vi "DiffDrivePoseEst_AddVisionMeasurement.vi"(9 "TImeStamp_Seconds":dbl=0.02, 10 "visionRobotPose":T10={"TRANSLATION"={"X"=0.0, "Y"=0.0}, "ROTATION"={"VALUE"=0.0, "COS"=1.0, "SIN"=0.0}} {"ROTATION"."SIN" format="%13.4f"; "ROTATION"."COS" format="%13.4f"; "ROTATION"."VALUE" format="%13.4f"; "TRANSLATION"."Y" format="%14.3f"; "TRANSLATION"."X" format="%14.3f"}, 11 "in DiffDrivePoseEstimate":T2={"M_VisionDiscR"=[], "m_nominal_dT"=0.0, "m_PrevTime_Sec"=0.0, "m_GyroOffset"={"VALUE"=0.0, "COS"=1.0, "SIN"=0.0}, "m_PrevAngle"={"VALUE"=0.0, "COS"=1.0, "SIN"=0.0}, "StartLeftEnc_M"=0.0, "StartRightEnc_M"=0.0, "m_Observer"={"m_P"=[], "m_xHat"=[], "States"=0, "Outputs"=0, "m_ContR"=[], "m_ContQ"=[], "m_SigmasF"=[], "m_dT_Sec"=0.0, "MERWE_SCALED_SIGMA_PTS"={"m_Wm"=[], "States"=0, "Alpha"=0.0, "m_Wc"=[], "Kappa"=0}, "meanFuncX"=refnum, "meanFuncY"=refnum, "residualFuncX"=refnum, "residualFuncY"=refnum, "addFuncX"=refnum, "addFuncXExtra"=variant, "residualFuncYExtra"=variant, "residualFuncXExtra"=variant, "MeanFuncYExtra"=variant, "MeanFuncXExtra"=variant, "Inputs"=0}, "m_latencyCompensator"={"m_pastObserverSnapshots "=[]}} {"m_PrevAngle"."SIN" format="%13.4f"; "m_PrevAngle"."COS" format="%13.4f"; "m_PrevAngle"."VALUE" format="%13.4f"; "m_GyroOffset"."SIN" format="%13.4f"; "m_GyroOffset"."COS" format="%13.4f"; "m_GyroOffset"."VALUE" format="%13.4f"}) -> (0 "Error":bool, 3 "Out DiffDrivePoseEstimate":T2={"M_VisionDiscR"=[], "m_nominal_dT"=0.0, "m_PrevTime_Sec"=0.0, "m_GyroOffset"={"VALUE"=0.0, "COS"=1.0, "SIN"=0.0}, "m_PrevAngle"={"VALUE"=0.0, "COS"=1.0, "SIN"=0.0}, "StartLeftEnc_M"=0.0, "StartRightEnc_M"=0.0, "m_Observer"={"m_P"=[], "m_xHat"=[], "States"=0, "Outputs"=0, "m_ContR"=[], "m_ContQ"=[], "m_SigmasF"=[], "m_dT_Sec"=0.0, "MERWE_SCALED_SIGMA_PTS"={"m_Wm"=[], "States"=0, "Alpha"=0.0, "m_Wc"=[], "Kappa"=0}, "meanFuncX"=refnum, "meanFuncY"=refnum, "residualFuncX"=refnum, "residualFuncY"=refnum, "addFuncX"=refnum, "addFuncXExtra"=variant, "residualFuncYExtra"=variant, "residualFuncXExtra"=variant, "MeanFuncYExtra"=variant, "MeanFuncXExtra"=variant, "Inputs"=0}, "m_latencyCompensator"={"m_pastObserverSnapshots "=[]}} {"m_PrevAngle"."SIN" format="%13.4f"; "m_PrevAngle"."COS" format="%13.4f"; "m_PrevAngle"."VALUE" format="%13.4f"; "m_GyroOffset"."SIN" format="%13.4f"; "m_GyroOffset"."COS" format="%13.4f"; "m_GyroOffset"."VALUE" format="%13.4f"})   [LabVIEW 2019, in "Trajectory_Library.lvlib"]
doc: "Add a vision measurement to the Unscented Kalman Filter. This will correct the odometry pose estimate while still accounting for measurement noise.\n \nThis method can be called as infrequently as you want, as long as you are calling DifferentialDrivePoseEstimator_update every loop.\n \nInputs:\n - InDIffDrivePoseEstimate -- Data cluster for this system\n - visionRobotPoseMeters -- The pose of the robot as measured by the vision camera.\n - timestampSeconds -- The timestamp of the vision measurement in seconds. Note that if you don't use your own time source by calling DifferentialDrivePoseEstimator_updateWithTime then you must use a timestamp with an epoch since FPGA startup (i.e. the epoch of this timestamp is the same epoch as Timer.getFPGATimestamp.) This means that you should use Timer.getFPGATimestamp as your time source in this case.\n\nOutputs:\n - OutDIffDrivePoseEstimate -- Data cluster for this system\n - Error -- Returns TRUE if an error occured."
uses:
  Trajectory_Library.lvlib
  DIFF_DRIVE_POSE_EST.ctl
  <vilib>/Analysis/Matrix/Datatypes/RealMatrix.ctl
  ROTATION2D.ctl
  UNSCENTED_KALMAN_FILTER.ctl
  MERWE_SCALED_SIGMA_PTS.ctl
  CALLBACK_FUNC_TYPE.ctl
  KALMAN_FILTER_LATENCY_COMP.ctl
  OBSERVER_SNAP_LIST_ITEM.ctl
  OBSERVER_SNAPSHOT.ctl
  POSE2D.ctl
  TRANSLATION2D.ctl
  VecBuilder_3x1Fill.vi
  Pose_getXYAngle.vi
  MatBuilder_Create.vi
  <vilib>/Analysis/Matrix/NI_Matrix.lvlib
panel:
  in  "Cluster":cluster{"VisionDiscreteR":T1}
  # "NOT A PARAMETER, JUST A DATA TYPE"
  # "<3, 3>"
  # "<Statess,1>"
  # "<States, States>"
  # "<Inputs, 1>"
  # "<Outputs,  1>"
  # "State Estimate <Statess,1>"
  # "<States, States>"
  # "<States, ?>"
  # "<Statess,  States>"
  # "<Outputs, Outputs>"
  # "<?, 1>"
  # "<?, 1>"
  # "<3, 3>"
  # "<Statess,1>"
  # "<States, States>"
  # "<Inputs, 1>"
  # "<Outputs,  1>"
  # "State Estimate <Statess,1>"
  # "<States, States>"
  # "<States, ?>"
  # "<Statess,  States>"
  # "<Outputs, Outputs>"
  # "<?, 1>"
  # "<?, 1>"
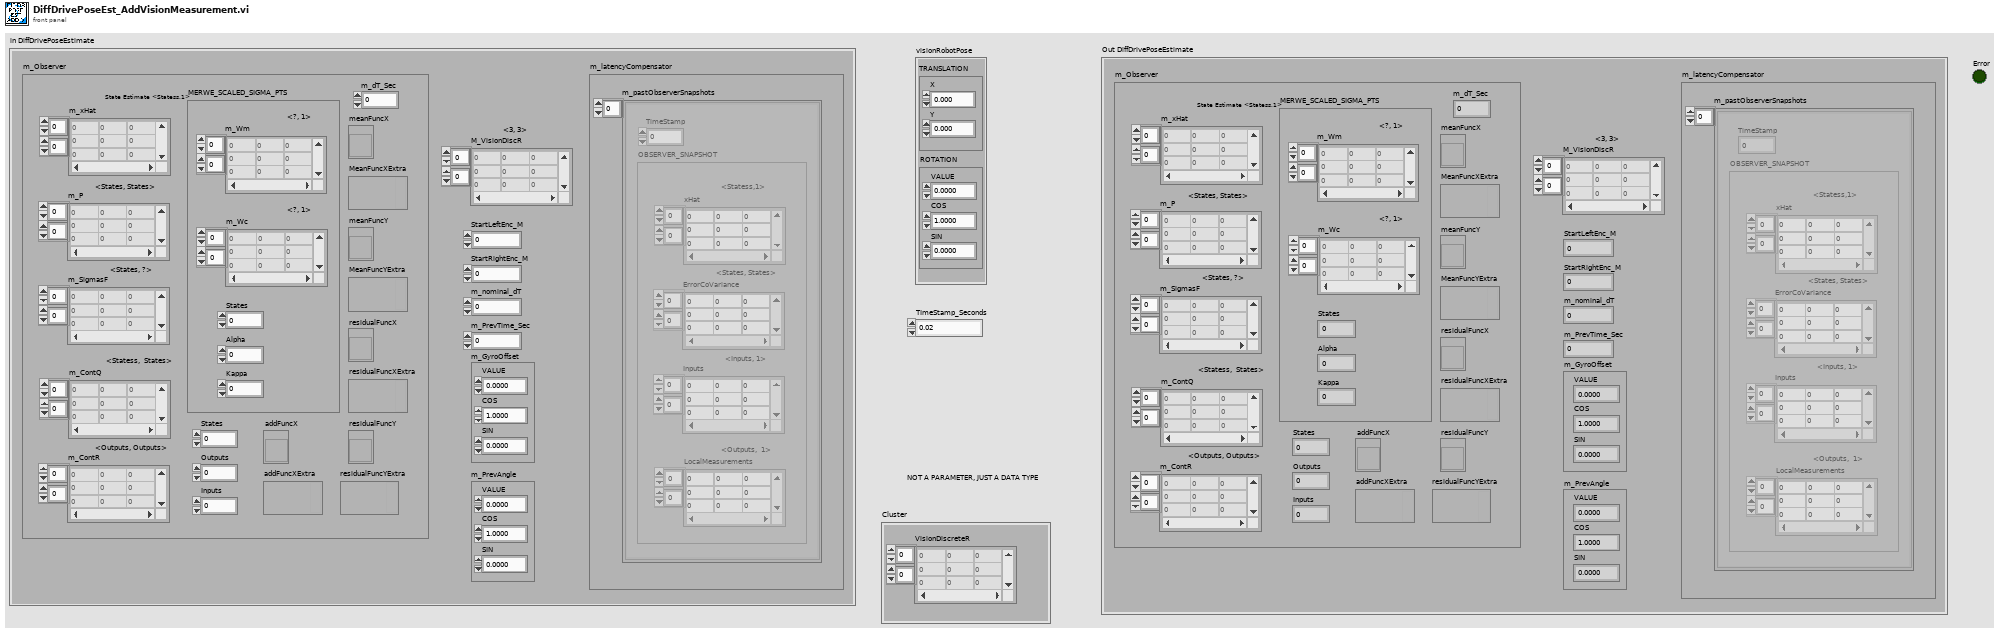
[diagram p1: front panel]
types:
  T1 = typedef "NI_Matrix.lvlib/RealMatrix.ctl" = dbl[][]
  T2 = typedef "Trajectory_Library.lvlib/DIFF_DRIVE_POSE_EST.ctl" = cluster{"M_VisionDiscR":T1, "m_nominal_dT":dbl, "m_PrevTime_Sec":dbl, "m_GyroOffset":T3, "m_PrevAngle":T3, "StartLeftEnc_M":dbl, "StartRightEnc_M":dbl, "m_Observer":T4, "m_latencyCompensator":T7}
  T3 = typedef "Trajectory_Library.lvlib/ROTATION2D.ctl" = cluster{"VALUE":dbl, "COS":dbl, "SIN":dbl}
  T4 = typedef "Trajectory_Library.lvlib/UNSCENTED_KALMAN_FILTER.ctl" = cluster{"m_P":T1, "m_xHat":T1, "States":i32, "Outputs":i32, "m_ContR":T1, "m_ContQ":T1, "m_SigmasF":T1, "m_dT_Sec":dbl, "MERWE_SCALED_SIGMA_PTS":T5, "meanFuncX":T6, "meanFuncY":T6, "residualFuncX":T6, "residualFuncY":T6, "addFuncX":T6, "addFuncXExtra":variant, "residualFuncYExtra":variant, "residualFuncXExtra":variant, "MeanFuncYExtra":variant, "MeanFuncXExtra":variant, "Inputs":i32}
  T5 = typedef "Trajectory_Library.lvlib/MERWE_SCALED_SIGMA_PTS.ctl" = cluster{"m_Wm":T1, "States":i32, "Alpha":dbl, "m_Wc":T1, "Kappa":i32}
  T6 = typedef "Trajectory_Library.lvlib/CALLBACK_FUNC_TYPE.ctl" = refnum<vi>
  T7 = typedef "Trajectory_Library.lvlib/KALMAN_FILTER_LATENCY_COMP.ctl" = cluster{"m_pastObserverSnapshots ":T8[]}
  T8 = typedef "Trajectory_Library.lvlib/OBSERVER_SNAP_LIST_ITEM.ctl" = cluster{"TimeStamp":dbl, "OBSERVER_SNAPSHOT":T9}
  T9 = typedef "Trajectory_Library.lvlib/OBSERVER_SNAPSHOT.ctl" = cluster{"ErrorCoVariance":T1, "xHat":T1, "LocalMeasurements":T1, "Inputs":T1}
  T10 = typedef "Trajectory_Library.lvlib/POSE2D.ctl" = cluster{"TRANSLATION":T11, "ROTATION":T3}
  T11 = typedef "Trajectory_Library.lvlib/TRANSLATION2D.ctl" = cluster{"X":dbl, "Y":dbl}
  T12 = typedef "Trajectory_Library.lvlib/KALMAN_FILTER_LATENCY_COMP_FUNC_GROUP.ctl" = cluster{"F_Func":T6, "H_Func":T6, "F_FuncExtra":variant, "H_FuncExtra":variant, "VisionCorrectExtra":variant, "VisionCorrect_Func":refnum<vi>}
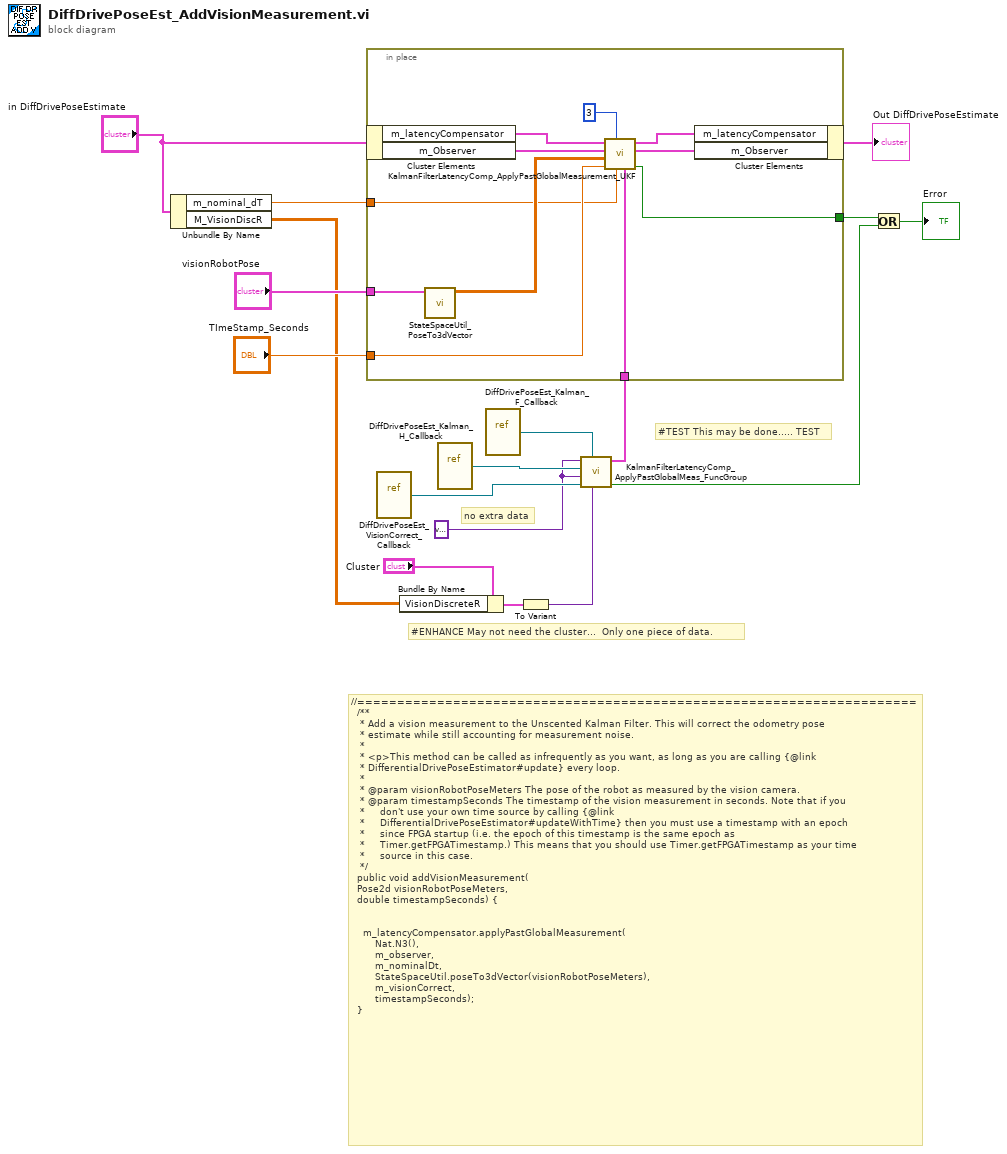
[diagram p0: block diagram]
diagram:
  w9 = variant ("ExtraData")
  # "#ENHANCE May not need the cluster...  Only one piece of data."
  # "no extra data"
  # "#TEST This may be done..... TEST"
  # "//======================================================================\n  /**\n   * Add a vision measurement to the Unscented Kalman Filter. This will correct the odometry pose\n   * estimate while still accounting for measurement noise.\n   *\n   * <p>This method can be called as infrequently as you want, as long as you are calling {@link\n   * DifferentialDrivePoseEstimator#update} every loop.\n   *\n   * @param visionRobotPoseMeters The pose of the robot as measured by the vision camera.\n   * @param timestampSeconds The timestamp of the vision measurement in seconds. Note that if you\n   *     don't use your own time source by calling {@link\n   *     DifferentialDrivePoseEstimator#updateWithTime} then you must use a timestamp with an epoch\n   *     since FPGA startup (i.e. the epoch of this timestamp is the same epoch as\n   *     Timer.getFPGATimestamp.) This means that you should use Timer.getFPGATimestamp as your time\n   *     source in this case.\n   */\n  public void addVisionMeasurement(\n\t\tPose2d visionRobotPoseMeters, \n\t\tdouble timestampSeconds) {\n\n\n    m_latencyCompensator.applyPastGlobalMeasurement(\n        Nat.N3(),\n        m_observer,\n        m_nominalDt,\n        StateSpaceUtil.poseTo3dVector(visionRobotPoseMeters),\n        m_visionCorrect,\n        timestampSeconds);\n  }"
  n1 = Unbundle By Name("in DiffDrivePoseEstimate") -> ("m_nominal_dT"=w13:dbl, "M_VisionDiscR"=w6:T1)
  n2 = vi-ref "DiffDrivePoseEst_VisionCorrect_Callback.vi"() -> (w10:refnum<vi>)
  n3 = Bundle By Name(cluster="Cluster", "VisionDiscreteR"=w6) -> (w5:cluster{"VisionDiscreteR":T1})
  n4 = vi-ref "DiffDrivePoseEst_Kalman_H_Callback.vi"() -> (w11:refnum<vi>)
  n5 = vi-ref "DiffDrivePoseEst_Kalman_F_Callback.vi"() -> (w12:refnum<vi>)
  n6 = To Variant(anything=w5) -> (Variant=w4:variant)
  n7 = call "KalmanFilterLatencyComp_ApplyPastGlobalMeas_FuncGroup.vi"("VisionCorrectExtra"=w4, "F_Func"=w12, "VisionCorrect_Func"=w10, "H_FuncExtra"=w9, "H_Func"=w11, "F_FuncExtra"=w9) -> ("Error"=w1:bool, "KALMAN_FILTER_LATENCY_COMP_FUNC_GROUP"=w8:T12)  [unwired: 4 in]
  n8 = in-place {
    in-place-border: "visionRobotPose" -> [w27]
    in-place-border: "TImeStamp_Seconds" -> [w25]
    in-place-border: w13 -> [w23]
    in-place-border: w8 -> [w22]
    in-place-border: [w18] -> w3
    n9 = in-place-cluster #1("in DiffDrivePoseEstimate") -> ("m_latencyCompensator"=w20:T7, "m_Observer"=w28:T4)
    n10 = call "StateSpaceUtil_PoseTo3dVector.vi"("Pose"=w27) -> ("Pose Vector"=w26:T1)  [unwired: 10 in]
    n11 = call "KalmanFilterLatencyComp_ApplyPastGlobalMeasurement_UKF.vi"("KALMAN_FILTER_LATENCY_COMP_FUNC_GROUP"=w22, "NominalDt_Sec"=w23, "Rows"=3, "TimeStamp_Sec"=w25, "Y"=w26, "in UNSCENTED_KALMAN_FILTER"=w28, "in KalmanFilterLatencyCompensator"=w20) -> ("Error"=w18:bool, "out UNSCENTED_KALMAN_FILTER"=w24:T4, "out KalmanFilterLatencyCompensator"=w19:T7)  [unwired: 2 in]
    n12 = in-place-cluster #1("m_latencyCompensator"=w19, "m_Observer"=w24) -> (→"Out DiffDrivePoseEstimate":T2)
  }
  n13 = Or(x=w3, y=w1) -> (x .or. y?=→"Error":bool)
